vi "niDTS WLAN OFDM Rx Test Get Documentation.vi"(0 "Dummy Test Handle in":T2, 11 "error in (no error)":errorcluster) -> (4 "Dummy Test Handle out":T2, 8 "Documentation":T1, 15 "error out":errorcluster)   [LabVIEW 2014, in "niDTS WLAN.lvlib"]
uses:
  niDTS WLAN.lvlib
  Rx Test/Includes/niDTS WLAN Rx Test INC Handle.ctl
  Rx Test/Objects/BASE_class/niDTS WLAN Rx Test.lvclass
  Framework/Test/Includes/niDTS Test INC Documentation.ctl
  Framework/niDTS Framework.lvlib
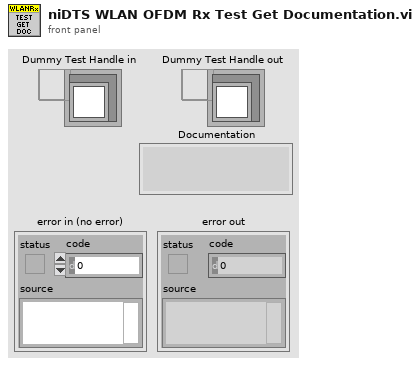
[diagram p1: front panel]
types:
  T1 = typedef "niDTS Framework.lvlib/niDTS Test INC Documentation.ctl" = string
  T2 = typedef "niDTS WLAN.lvlib/niDTS WLAN Rx Test INC Handle.ctl" = refnum<data-value>
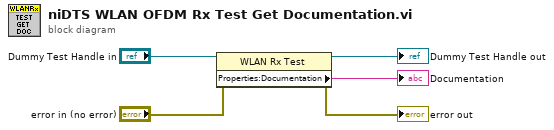
[diagram p0: block diagram]
diagram:
  n1 = property class="WLAN Rx Test"(reference="Dummy Test Handle in", error in="error in (no error)") -> (reference out=→"Dummy Test Handle out":T2, error out=→"error out":errorcluster, "Properties:Documentation"=→"Documentation":T1)
